vi "EDIT ITEM IN PGSQL.vi"(9 "USER/ITEM DATA TRANSFER":T1(array[cluster]), 10 "ITEM DATA IN":T2) -> (2 "ITEM DATA OUT":T2)   [LabVIEW 2019]
uses:
  Controls/Column Names/Inventory Column Names.ctl
  <vilib>/addons/database/Connection.llb/DB Tools Open Connec (String).vi
  <vilib>/addons/database/NI_Database_API.lvlib
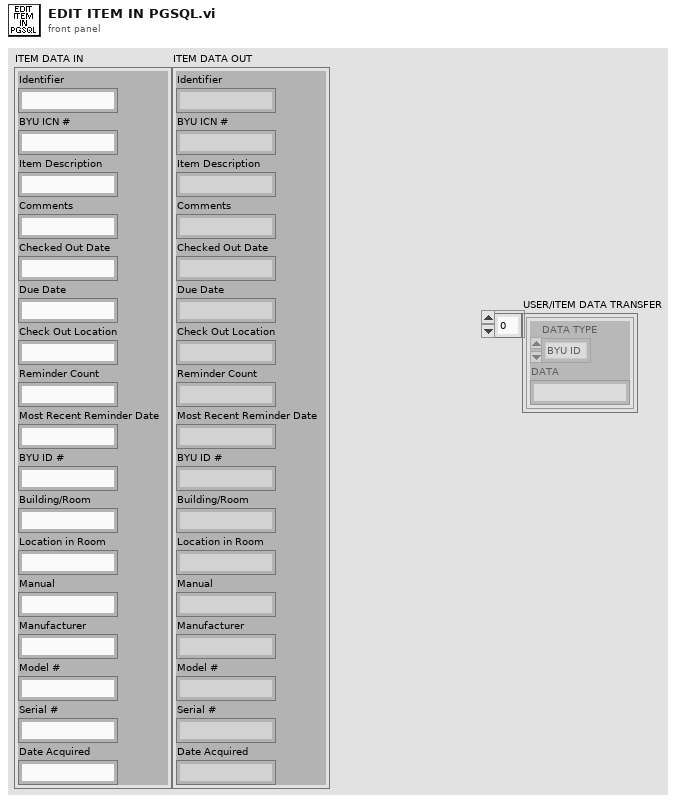
[diagram p1: front panel]
types:
  T1 = cluster{"DATA TYPE":enum16{"BYU ID", "ME#/IDENTIFIER", "BYU ICN"}, "DATA":string}[]
  T2 = cluster{"Identifier":string, "BYU ICN #":string, "Item Description":string, "Comments":string, "Checked Out Date":string, "Due Date":string, "Check Out Location":string, "Reminder Count":string, "Most Recent Reminder Date":string, "BYU ID #":string, "Building/Room":string, "Location in Room":string, "Manual":string, "Manufacturer":string, "Model #":string, "Serial #":string, "Date Acquired":string}
  T3 = typedef "Inventory Column Names.ctl" = string[]
  T4 = cluster{"DATA TYPE":enum16{"BYU ID", "ME#/IDENTIFIER", "BYU ICN"}, "DATA":string}
  T5 = typedef "NI_Database_API.lvlib/Conn ObjectReference.ctl" = refnum<k1>
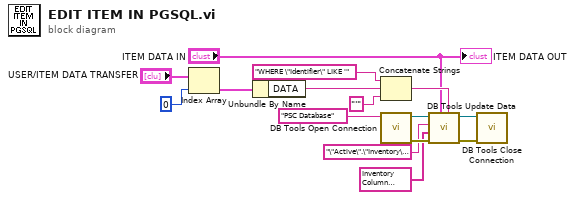
[diagram p0: block diagram]
diagram:
  n1 = Index Array(array="USER/ITEM DATA TRANSFER", index=0) -> (element=w1:T4)
  n2 = Unbundle By Name(w1) -> ("DATA"=w15:string)
  n3 = Concatenate Strings("WHERE \"Identifier\" LIKE '" ("string"), w15, "'" ("string")) -> (w12:string)
  n4 = call-poly <vilib>:"DB Tools Open Connection.vi"("connection information"="PSC Database" ("string")) -> ("error out"=w13:errorcluster, "connection reference"=w14:T5)  [unwired: 7 in]
  n5 = call <vilib>:"DB Tools Update Data.vi"("condition"=w12, "data"="ITEM DATA IN", "error in (no error)"=w13, "columns"=T3 ["\"Identifier\"", "\"BYU ICN #\"", "\"Item Description\"", "\"Comments\"", "\"Checked Out Date\"", "\"Due Date\"", "\"Check Out Location\"", "\"Reminder Count\"", "\"Most Recent Reminder Date\"", "\"BYU ID #\"", "\"Building/Room\"", "\"Location in Room\"", "\"Manual\"", "\"Manufacturer\"", "\"Model #\"", "\"Serial #\"", "\"Date Acquired\""] ("INVENTORY COLUMN NAMES"), "table"="\"Active\".\"Inventory\" ", "connection reference"=w14) -> ("error out"=w10:errorcluster, "connection reference out"=w11:T5)  [unwired: 4 in]
  n6 = call <vilib>:"DB Tools Close Connection.vi"("error in (no error)"=w10, "connection reference"=w11) -> ()  [unwired: 5 in, 1 out]
  "ITEM DATA OUT" <- "ITEM DATA IN"
